vi "MulliganFilenumber.vi"(4 "error in (no error)":errorcluster, 6 "FileNumber":string, 7 "SequenceHistory ref":refnum<vi>) -> (0 "error out":errorcluster, 1 "Success":bool, 3 "SequenceHistory ref out":refnum<vi>)   [LabVIEW 2013]
doc: "Does a Mulligan on the requested FileNumber, if found in the Sequence History Table"
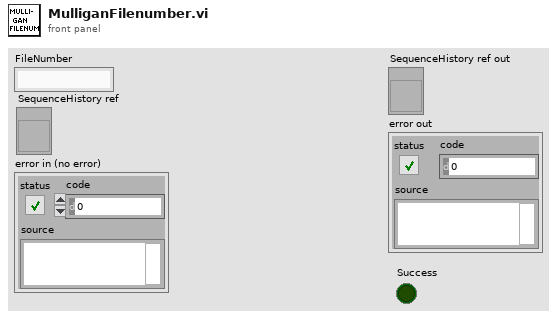
[diagram p1: front panel]
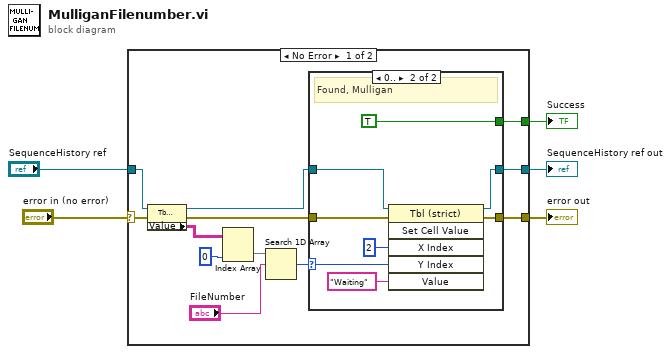
[diagram p0: block diagram]
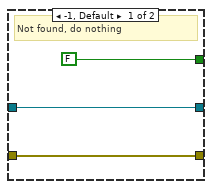
[diagram p2: hidden frame]
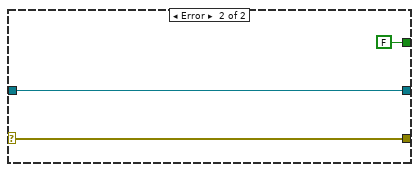
[diagram p3: hidden frame]
diagram:
  n1 = case shown="No Error" "error in (no error)" {
    selector: "error in (no error)" -> [w8 w31]
    tunnel: [w10 w30] -> w5
    tunnel: [w9 w31] -> w4
    tunnel: "SequenceHistory ref" -> [w7 w30]
    tunnel: [w6 FALSE] -> w1
    frame No Error {
      n2 = property on="Property Node" class="Tbl (strict)"(reference=w7, error in=w8) -> (reference out=w12:refnum<vi>, error out=w13:errorcluster, "Value"=w17:string[][])
      n3 = Index Array(array=w17, index (col)=0 ("disabled index (col)")) -> (element=w15:string[])  [unwired: 1 in]
      n4 = Search 1D Array(1D array=w15, element="FileNumber") -> (index of element=w14:i32)  [unwired: 1 in]
      n5 = case shown="0.." w14 {
        selector: w14 -> [_ w28]
        tunnel: w13 -> [w19 w25]
        tunnel: w12 -> [w20 w24]
        tunnel: [w20 w23] -> w10
        tunnel: [w19 w22] -> w9
        tunnel: [FALSE TRUE] -> w6
        frame -1, Default {
          # "Not found, do nothing"
        }
        frame 0.. {
          # "Found, Mulligan"
          n6 = invoke on="Invoke Node" class="Tbl (strict)" method="Set Cell Value"(reference=w24, error in=w25, "X Index"=2, "Y Index"=w28, "Value"="Waiting") -> (reference out=w23:refnum<vi>, error out=w22:errorcluster)  [unwired: 1 in, 4 out]
        }
      }
    }
    frame Error {
    }
  }
  "SequenceHistory ref out" <- w5
  "error out" <- w4
  "Success" <- w1
